vi "Temp.vi"() -> (0 "Temp":dbl)   [LabVIEW 2015]
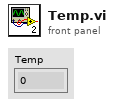
[diagram p1: front panel]
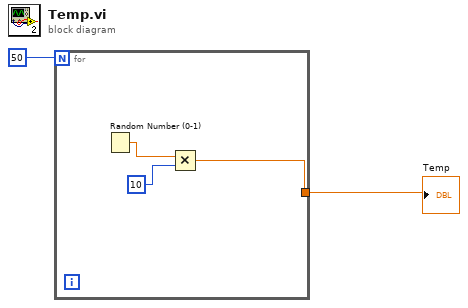
[diagram p0: block diagram]
diagram:
  n1 = for {
    N: 50 -> [_]
    tunnel: [w4] -> w1
    n2 = Random Number (0-1) ("Random Number (1-10)")() -> (number: 0 to 1=w5:dbl)
    n3 = Multiply(x=w5, y=10) -> (x*y=w4:dbl)
  }
  "Temp" <- w1
